vi "setMeasurement2450.vi"(1 "Measure":T1) -> (0 "String":string)   [LabVIEW 2021]
uses:
  Measure2450.ctl
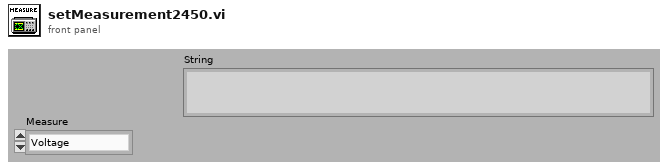
[diagram p1: front panel]
types:
  T1 = typedef "Measure2450.ctl" = enum16{"Voltage", "Current"}
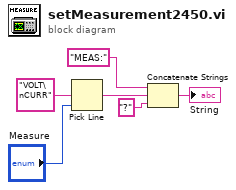
[diagram p0: block diagram]
diagram:
  n1 = Pick Line(multi-line string="VOLT\nCURR", line index="Measure") -> (output string=w2:string)  [unwired: 1 in]
  n2 = Concatenate Strings("MEAS:", w2, "?") -> (→"String":string)
